vi "Constructor.vi"(8 "error in":errorcluster, 9 "Value":i32, 10 "Name":string, 11 "Int in":refnum<class "Int.lvclass">) -> (0 "error out":errorcluster, 3 "Int out":refnum<class "Int.lvclass">)   [LabVIEW 2021, in "ProligentXMLGenerator.lvlib" / "Int.lvclass"]
uses:
  Int.lvclass
  Int.lvclass/Int.ctl
  Attribute/Attribute.lvclass
  C:/Projects/proligent-xml-generator-labview/src/ProligentXMLGenerator/Base/Attribute/Attribute.lvclass
  C:/Projects/proligent-xml-generator-labview/src/ProligentXMLGenerator/Base/Int/Int.lvclass
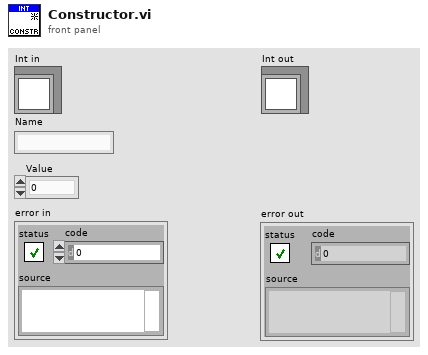
[diagram p1: front panel]
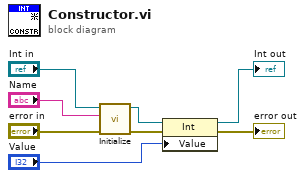
[diagram p0: block diagram]
diagram:
  n1 = call "Initialize.vi"("error in"="error in", "Name"="Name", "Attribute in"="Int in") -> ("error out"=w4:errorcluster, "Attribute out"=w3:refnum<class "Int.lvclass">)  [unwired: 7 in]
  n2 = property on="Property Node" class="Int"(reference=w3, error in=w4, "Value"="Value") -> (reference out=→"Int out":refnum<class "Int.lvclass">, error out=→"error out":errorcluster)
